vi "Get VS Amplitude From String.vi"(8 "error in (no error)":errorcluster, 10 "index":i32, 11 "text":string) -> (0 "error out":errorcluster, 1 "function return":u32, 2 "index out":i32, 3 "text out":string)   [LabVIEW 2014, in "atmcd32d.lvlib"]
doc: "unsigned int WINAPI GetVSAmplitudeFromString(char * text, int * index);"
uses:
  atmcd32d.lvlib
  atmcd32d.dll
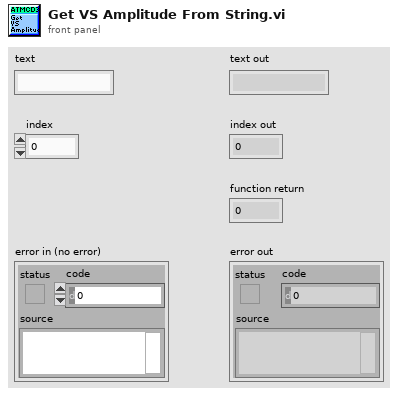
[diagram p1: front panel]
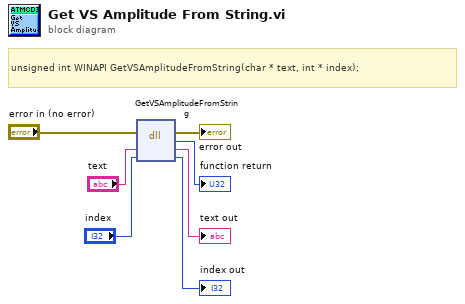
[diagram p0: block diagram]
diagram:
  # "unsigned int WINAPI GetVSAmplitudeFromString(char * text, int * index);"
  n1 = dll-call lib="C:/Users/Bakir/Documents/Lambda2-Testing/lib/Andorlib/atmcd32d.*" fn="GetVSAmplitudeFromString"(error in="error in (no error)", "text"="text", "index"="index") -> (error out=→"error out":errorcluster, →"function return":u32, "text"=→"text out":string, "index"=→"index out":i32)  [unwired: 2 in, 1 out]
